vi "Max_Min_Limiter.vi"(2 "Analysis info":T2={"Colour"=0, "Inst type"=enum."Pitot-static tube", "Inst name"="Manometer voltage", "Symbol"="U", "Code name"="", "Extra Info"="U", "Inst Array"=enum."PWA", "Extra Titles"=[], "Extra Values"=[], "U"=0.0, "u^2"=0.0, "u^3"=0.0, "u^4"=0.0, "Skew_u"=0.0, "Kurt_u"=0.0, "Sd Error in Mean"=0.0, "% u'/U"=0.0, "X"=0.0, "Y"=0.0, "Z"=0.0, "Timescale integral Estimate"=0.0, "Sd Error in Variance"=0.0, "Calib File"=path "", "Calib Constants"=[], "Output Position"=FALSE, "Full Stats"=FALSE, "Av Sampling Rate"=0.0, "Av No of Samples"=0.0, "Total Meas Time (s)"=0.0, "ADAM Ch Name"="", "Max value"=0.0, "Min value"=0.0, "Sync Delay Time (s)"=0.0} {"Sync Delay Time (s)" format="%.2f"; "Sd Error in Variance" format="%.2f"; "Skew_u" format="%.2f"; "% u'/U" format="%.2f"; "Sd Error in Mean" format="%.2f"; "Kurt_u" format="%.2f"; "u^4" format="%.2f"; "u^3" format="%.2f"; "U" format="%.2f"; "u^2" format="%.2f"}, 3 "Time Trace In":T1) -> (1 "Time Trace Out":T1)   [LabVIEW 2017]
uses:
  Controls/Analysis_info_cluster.ctl
  Controls/Inst_type.ctl
  Controls/Instrument_Array.ctl
  Controls/Time_Trace_Cluster.ctl
  Controls/Post_Process.ctl
  Globals/Meas_global.vi
  <vilib>/Analysis/NI_AALBase.lvlib
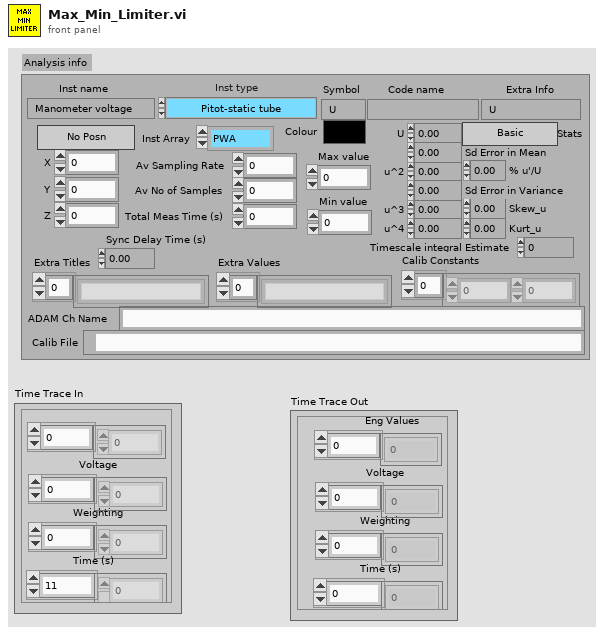
[diagram p1: front panel]
types:
  T1 = typedef "Time_Trace_Cluster.ctl" = cluster{"Weighting":dbl[], "Time (s)":dbl[], "Voltage":dbl[], "Eng Values":dbl[]}
  T2 = typedef "Analysis_info_cluster.ctl" = cluster{"Colour":u32, "Inst type":T3, "Inst name":string, "Symbol":string, "Code name":string, "Extra Info":string, "Inst Array":T4, "Extra Titles":string[], "Extra Values":string[], "U":dbl, "u^2":dbl, "u^3":dbl, "u^4":dbl, "Skew_u":dbl, "Kurt_u":dbl, "Sd Error in Mean":dbl, "% u'/U":dbl, "X":dbl, "Y":dbl, "Z":dbl, "Timescale integral Estimate":dbl, "Sd Error in Variance":dbl, "Calib File":path, "Calib Constants":dbl[], "Output Position":bool, "Full Stats":bool, "Av Sampling Rate":dbl, "Av No of Samples":dbl, "Total Meas Time (s)":dbl, "ADAM Ch Name":string, "Max value":dbl, "Min value":dbl, "Sync Delay Time (s)":dbl}
  T3 = typedef "Inst_type.ctl" = enum16{"Propeller anemometer", "Raw voltage", "Pressure Transducer", "Pitot-static tube", "Preston tube", "Hot wire", "Cross wire 1", "Cross wire 2", "Generic Linear", "Generic Polynomial", "Generic BackPoly", "Fast FID", "Thermocouple", "Cold wire", "Pulsed Wire", "LDA Vel", "LDA Tran time", "LDA Arr time", "Microphone"}
  T4 = typedef "Instrument_Array.ctl" = enum16{"PWA", "LDA", "Analogue"}
  T5 = typedef "Post_Process.ctl" = enum16{"Take New Data", "Post Process Raw Data File"}
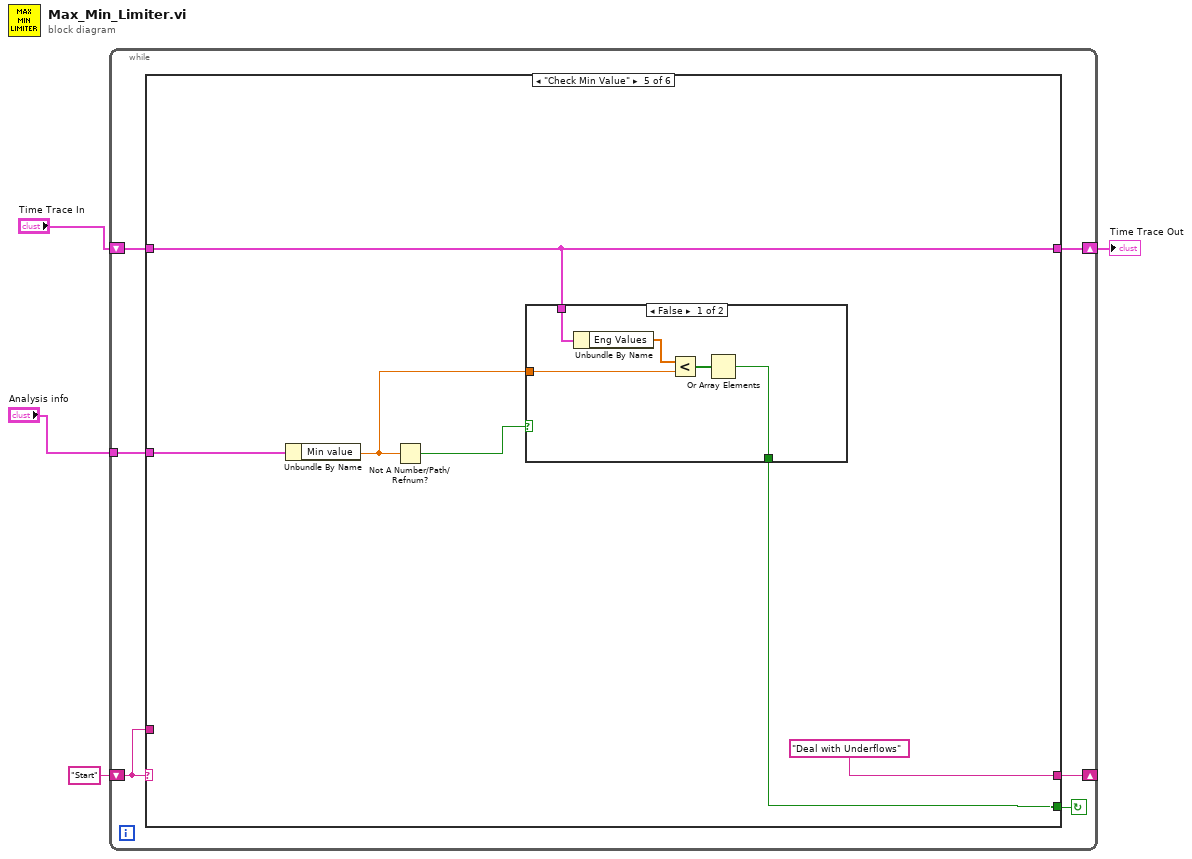
[diagram p0: block diagram]
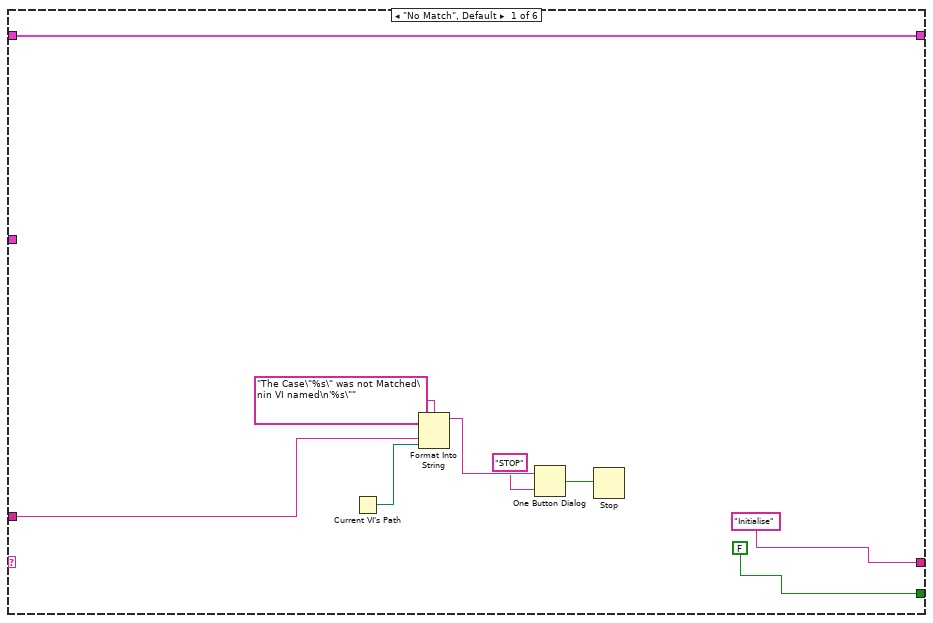
[diagram p2: hidden frame]
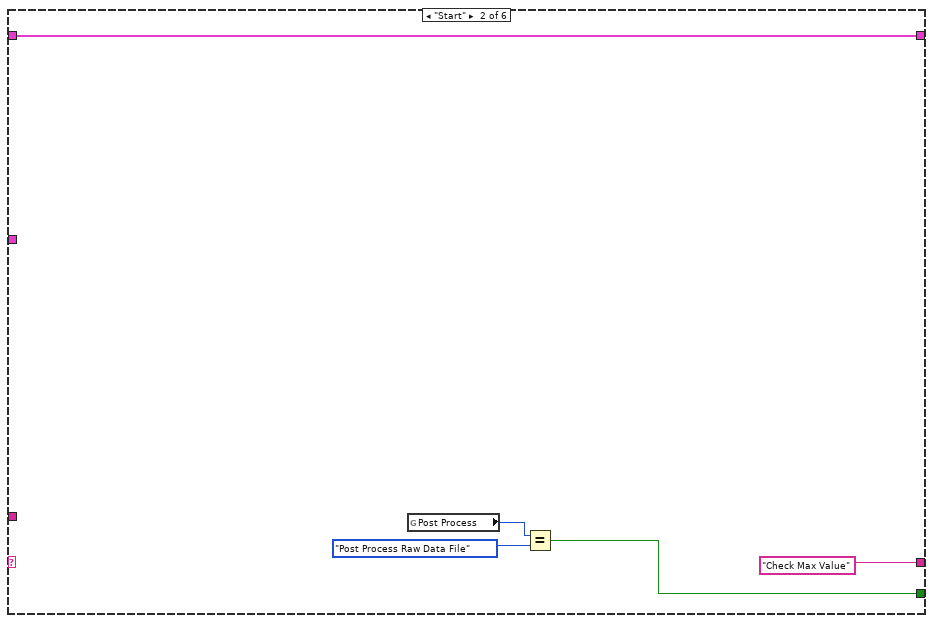
[diagram p3: hidden frame]
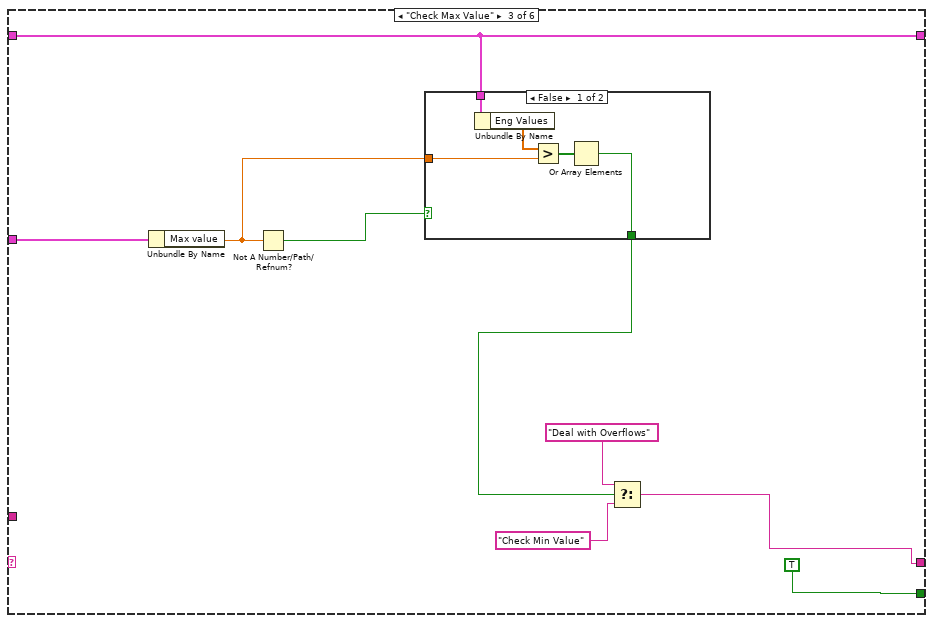
[diagram p4: hidden frame]
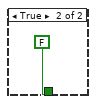
[diagram p5: hidden frame]
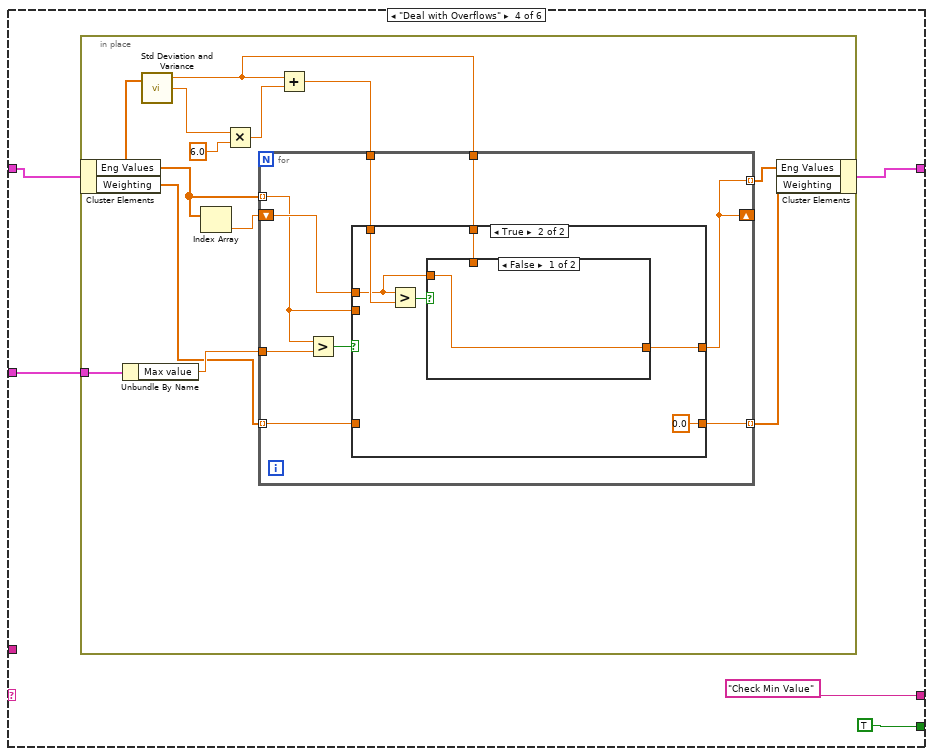
[diagram p6: hidden frame]
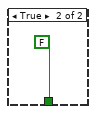
[diagram p9: hidden frame]
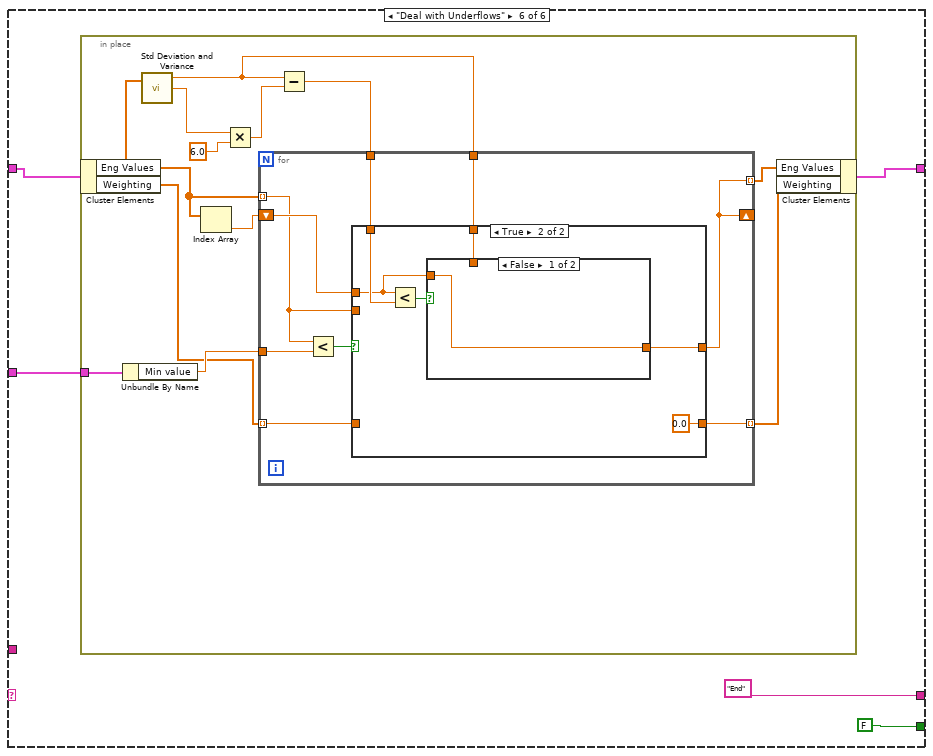
[diagram p10: hidden frame]
diagram:
  n1 = while {
    shift-left: "Start" ("f") -> [w8]
    shift-right: [w9] -> _
    tunnel: "Analysis info" -> [w7]
    shift-right: [w5] -> w2
    shift-left: "Time Trace In" -> [w6]
    stop <- w10 continue-if-true
    n2 = case shown="\"Check Min Value\"" w8 {
      tunnel: [FALSE w21 TRUE TRUE w77 FALSE] -> w10
      tunnel: ["Initialise" "Check Max Value" w31 "Check Min Value" "Deal with Underflows" ("f") "End"] -> w9
      tunnel: w8 -> [w14 _ _ _ _ _]
      tunnel: w7 -> [_ _ w32 w42 w81 w90]
      tunnel: w6 -> [w11 w20 w25 w41 w76 w89]
      tunnel: [w11 w20 w25 w40 w76 w88] -> w5
      frame "No Match", Default {
        n3 = Current VI's Path() -> (path=w13:path)
        n4 = Format Into String(format string="The Case\"%s\" was not Matched\nin VI named\n'%s\"" ("Format String"), w14, w13) -> (resulting string=w17:string)  [unwired: 2 in, 1 out]
        n5 = One Button Dialog(message=w17, button name ("OK")="STOP") -> (true=w15:bool)
        n6 = Stop(stop? (T)=w15) -> ()
      }
      frame "Start" {
        n7 = global read "Meas_global.vi" "Post Process"() -> (w22:T5)
        n8 = Equal?(x=w22, y=Post_Process."Post Process Raw Data File" ("Post Process")) -> (x = y?=w21:bool)
      }
      frame "Check Max Value" {
        n9 = Unbundle By Name(w32) -> ("Max value"=w29:dbl)
        n10 = Not A Number/Path/Refnum?(number/path/refnum=w29) -> (NaN/Path/Refnum?=w30:bool)
        n11 = case shown="False" w30 {
          tunnel: w25 -> [w36 _]
          tunnel: w29 -> [w38 _]
          tunnel: [w37 FALSE] -> w28
          frame False {
            n12 = Unbundle By Name(w36) -> ("Eng Values"=w35:dbl[])
            n13 = Greater?(x=w35, y=w38) -> (0:w34:bool[])
            n14 = Or Array Elements(Boolean array=w34) -> (logical OR=w37:bool)
          }
          frame True {
          }
        }
        n15 = Select(t="Deal with Overflows" ("f"), s=w28, f="Check Min Value") -> (s? t:f=w31:string)
      }
      frame "Deal with Overflows" {
        n16 = in-place {
          in-place-border: w42 -> [w56]
          n17 = in-place-cluster #1(w41) -> ("Eng Values"=w48:dbl[], "Weighting"=w47:dbl[])
          n18 = Unbundle By Name(w56) -> ("Max value"=w55:dbl)
          n19 = call <vilib>:"Std Deviation and Variance.vi"("X"=w48) -> ("mean"=w49:dbl, "standard deviation"=w53:dbl)  [unwired: 1 in, 1 out]
          n20 = Index Array(array=w48) -> (element=w54:dbl)  [unwired: 1 in]
          n21 = Multiply(x=w53, y=6.0) -> (x*y=w51:dbl)
          n22 = Add(x=w49, y=w51) -> (x+y=w50:dbl)
          n23 = for {
            tunnel: w48 -> [w60] mode=indexing
            tunnel: w55 -> [w65]
            shift-right: [w59] -> _
            shift-left: w54 -> [w63]
            tunnel: w50 -> [w62]
            tunnel: w49 -> [w61]
            tunnel: [w59] -> w46 mode=indexing
            tunnel: [w58] -> w45 mode=indexing
            tunnel: w47 -> [w57] mode=indexing
            n24 = Greater?(x=w60, y=w65) -> (0:w64:bool)
            n25 = case shown="True" w64 {
              tunnel: w63 -> [_ w69]
              tunnel: w62 -> [_ w73]
              tunnel: [w67 w71] -> w59
              tunnel: w61 -> [_ w70]
              tunnel: w60 -> [w67 _]
              tunnel: [w66 0.0 ("Numeric")] -> w58
              tunnel: w57 -> [w66 _]
              frame False {
              }
              frame True {
                n26 = Greater?(x=w69, y=w73) -> (0:w72:bool)
                n27 = case shown="False" w72 {
                  tunnel: [w74 w75] -> w71
                  tunnel: w70 -> [_ w75]
                  tunnel: w69 -> [w74 _]
                  frame False {
                  }
                  frame True {
                  }
                }
              }
            }
          }
          n28 = in-place-cluster #1("Eng Values"=w46, "Weighting"=w45) -> (w40:T1)
        }
      }
      frame "Check Min Value" {
        n29 = Unbundle By Name(w81) -> ("Min value"=w79:dbl)
        n30 = Not A Number/Path/Refnum?(number/path/refnum=w79) -> (NaN/Path/Refnum?=w80:bool)
        n31 = case shown="False" w80 {
          tunnel: w76 -> [w84 _]
          tunnel: w79 -> [w86 _]
          tunnel: [w85 FALSE] -> w77
          frame False {
            n32 = Unbundle By Name(w84) -> ("Eng Values"=w83:dbl[])
            n33 = Less?(x=w83, y=w86) -> (x < y?=w82:bool[])
            n34 = Or Array Elements(Boolean array=w82) -> (logical OR=w85:bool)
          }
          frame True {
          }
        }
      }
      frame "Deal with Underflows" {
        n35 = in-place {
          in-place-border: w90 -> [w104]
          n36 = in-place-cluster #2(w89) -> ("Eng Values"=w96:dbl[], "Weighting"=w95:dbl[])
          n37 = Unbundle By Name(w104) -> ("Min value"=w103:dbl)
          n38 = call <vilib>:"Std Deviation and Variance.vi"("X"=w96) -> ("mean"=w97:dbl, "standard deviation"=w101:dbl)  [unwired: 1 in, 1 out]
          n39 = Index Array(array=w96) -> (element=w102:dbl)  [unwired: 1 in]
          n40 = Multiply(x=w101, y=6.0) -> (x*y=w99:dbl)
          n41 = Subtract(x=w97, y=w99) -> (x-y=w98:dbl)
          n42 = for {
            tunnel: w96 -> [w108] mode=indexing
            tunnel: w103 -> [w113]
            shift-right: [w107] -> _
            shift-left: w102 -> [w111]
            tunnel: w98 -> [w110]
            tunnel: w97 -> [w109]
            tunnel: [w107] -> w94 mode=indexing
            tunnel: [w106] -> w93 mode=indexing
            tunnel: w95 -> [w105] mode=indexing
            n43 = Less?(x=w108, y=w113) -> (x < y?=w112:bool)
            n44 = case shown="True" w112 {
              tunnel: w111 -> [_ w117]
              tunnel: w110 -> [_ w121]
              tunnel: [w115 w119] -> w107
              tunnel: w109 -> [_ w118]
              tunnel: w108 -> [w115 _]
              tunnel: [w114 0.0 ("Numeric")] -> w106
              tunnel: w105 -> [w114 _]
              frame False {
              }
              frame True {
                n45 = Less?(x=w117, y=w121) -> (x < y?=w120:bool)
                n46 = case shown="False" w120 {
                  tunnel: [w122 w123] -> w119
                  tunnel: w118 -> [_ w123]
                  tunnel: w117 -> [w122 _]
                  frame False {
                  }
                  frame True {
                  }
                }
              }
            }
          }
          n47 = in-place-cluster #2("Eng Values"=w94, "Weighting"=w93) -> (w88:T1)
        }
      }
    }
  }
  "Time Trace Out" <- w2
